vi "Asia set maximum flowrate (SubVI).vi"(11 "Syringe Diam":sgl) -> (3 "Max Flowrate":sgl)   [LabVIEW 2018]
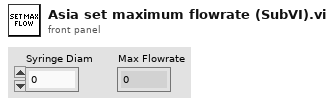
[diagram p1: front panel]
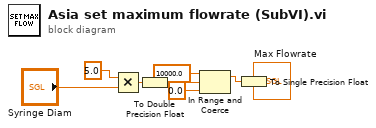
[diagram p0: block diagram]
diagram:
  n1 = Multiply(x=sgl 5.0, y="Syringe Diam") -> (x*y=w6:sgl)
  n2 = To Double Precision Float(number=w6) -> (double precision float=w3:dbl)
  n3 = In Range and Coerce(upper limit=10000.0, x=w3, lower limit=0.0) -> (coerced(x)=w4:dbl)  [unwired: 1 out]
  n4 = To Single Precision Float(number=w4) -> (single precision float=→"Max Flowrate":sgl)
